vi "GVSWait Graph Close.vi"(10 "vi reference":refnum<vi>) -> ()   [LabVIEW 2013]
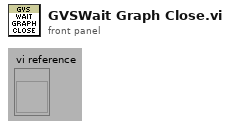
[diagram p1: front panel]
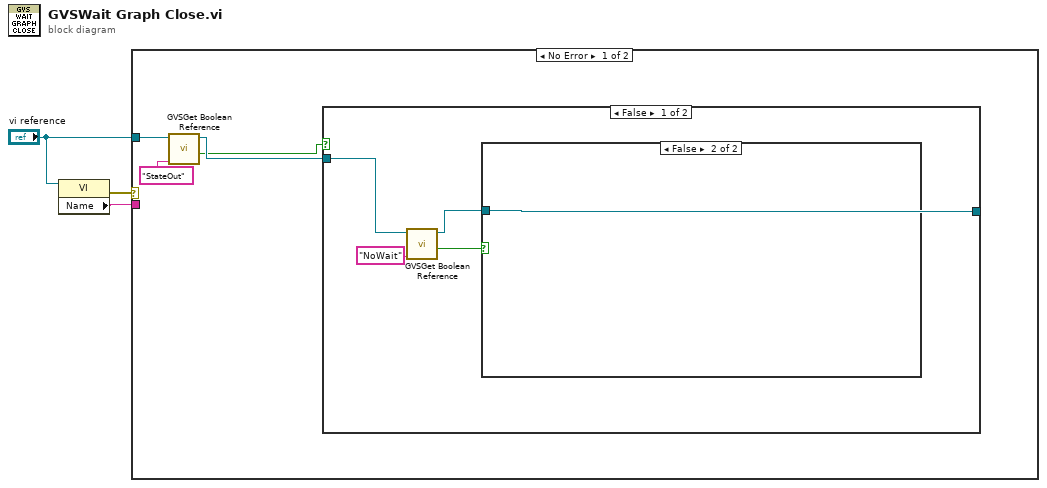
[diagram p0: block diagram]
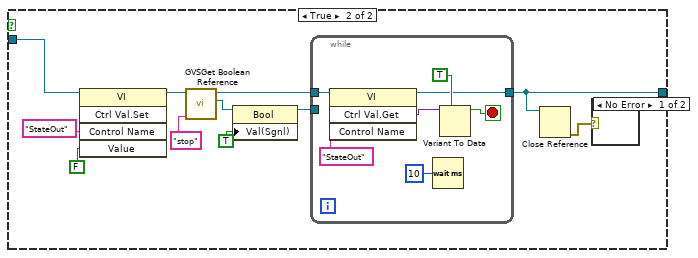
[diagram p3: hidden frame]
diagram:
  n1 = property class="VI"(reference="vi reference") -> (error out=w3:errorcluster, "Name"=w1:string)  [unwired: 1 in, 1 out]
  n2 = case shown="No Error" w3 {
    tunnel: "vi reference" -> [w6 _]
    tunnel: w1 -> [_ _]
    frame No Error {
      n3 = call "GVSGet Boolean Reference.vi"("Label Name"="StateOut", "VI Refnum"=w6) -> ("Boolean"=w4:bool, "VI Refnum Out"=w5:refnum<vi>)  [unwired: 7 in, 1 out]
      n4 = case shown="False" w4 {
        tunnel: w5 -> [w10 w15]
        tunnel: [w9 w13] -> _
        frame False {
          n5 = call "GVSGet Boolean Reference.vi"("Label Name"="NoWait", "VI Refnum"=w10) -> ("Boolean"=w8:bool, "VI Refnum Out"=w9:refnum<vi>)  [unwired: 7 in, 1 out]
          n6 = case shown="False" w8 {
            tunnel: w9 -> [_ _]
            frame True {
            }
            frame False {
            }
          }
        }
        frame True {
          n7 = invoke class="VI" method="Ctrl Val.Set"(reference=w15, "Control Name"="StateOut", "Value"=FALSE) -> (reference out=w17:refnum<vi>)  [unwired: 2 in, 4 out]
          n8 = call "GVSGet Boolean Reference.vi"("Label Name"="stop", "VI Refnum"=w17) -> ("Boolean Ref"=w20:refnum<vi>, "VI Refnum Out"=w16:refnum<vi>)  [unwired: 7 in, 1 out]
          n9 = property class="Bool"(reference=w20, "Val(Sgnl)"=TRUE) -> (reference out=w14:refnum<vi>)  [unwired: 1 in, 1 out]
          n10 = while {
            tunnel: w16 -> [w28]
            tunnel: [w24] -> w13
            tunnel: w14 -> [_]
            stop <- w25 stop-if-true
            n11 = invoke class="VI" method="Ctrl Val.Get"(reference=w28, "Control Name"="StateOut") -> (reference out=w24:refnum<vi>, "Get Control Value Variant"=w27:variant)  [unwired: 2 in, 2 out]
            n12 = Wait (ms)(milliseconds to wait=u32 10) -> ()  [unwired: 1 out]
            n13 = Variant To Data(type=TRUE, Variant=w27) -> (data=w25:bool)  [unwired: 1 in, 1 out]
          }
          n14 = Close Reference(reference=w13) -> (error out=w12:errorcluster)  [unwired: 1 in]
          n15 = case shown="No Error" w12 {
            frame No Error {
            }
            frame Error {
            }
          }
        }
      }
    }
    frame Error {
    }
  }
